vi "VI Konfig LAMBDA.vi"() -> ()   [LabVIEW 2020, in "Lambda_ Komm.lvlib"]
uses:
  Lambda_ Komm.lvlib
  CalGas Aufschaltung/Aufschaltung CalGas_ANZEIGE.ctl
  Visualisierungs Elemente/Auswahlfeld.ctl
  Visualisierungs Elemente/Zahlen-Ausgabefeld.ctl
  CalGas Aufschaltung/FGV CalGas Aktionen.ctl
  FT-IR/FGV FT-IR Gasliste Aktionen.ctl
  FGV Status Lambda Aktionen.ctl
  Messdaten/Aktionen FGV Messdaten.ctl
  FT-IR/FGV FT-IR Parameter.vi
  CalGas Aufschaltung/CalGas Aufschaltung.lvlib
  Grafik/Grafik.lvlib
  FT-IR/FT-IR.lvlib
  Allgemein/allgemeine Sub-VIs.lvlib
  Messdaten/Messdaten.lvlib
panel:
  out "Mwert 3":sgl format="%.1f"
  out "PMwert 3":sgl format="%.1f"
  out "Mwert 2":sgl format="%.3f"
  out "PMwert 2":sgl format="%.3f"
  out "Mwert":sgl format="%.1f"
  out "PMwert":sgl format="%.1f"
  out "A/F Messwertfehler:":bool
  out "O2 Messwertfehler:":bool
  out "Sonden-Innenwiderstand Fehler:":bool
  out "Lambda Messwertfehler:":bool
  out "Kommunikationsfehler:":bool
  out "Sonden-Innenwiderstand:":T1 caption="Ohm" format="%#_5g"
  out "A/F":string
  out "Wert A/F":T1 caption="Konzentration" format="%.1f"
  out "O2":string
  out "Lambda":string
  out "Wert O2":T1 caption="Konzentration" format="%.3f"
  out "Wert Lambda":T1 caption="Konzentration" format="%.1f"
  in  "Aufschaltung CalGas":T2 {"Analysator" items=["FT-IR", "NDIR CO2", "NDIR CO", "PMA", "FID", "CLD"]; "Aufschaltpunkt" items=["über Filterblock", "Analysator direkt", "über Gasteiler", "Gasteiler Eingang"]; "Kalibriergas" items=["Stickstoff", "---", "---", "NOx lo", "NOx hi", "---", "CO2", "CO", "---", "O2", "---", "HC", "---"]}
  out "Graph 3":waveform(dbl)[](graph)
  out "Graph 2":waveform(dbl)[](graph)
  out "Graph1":waveform(dbl)[](graph)
  # "Konfig LAMBDA"
  # "Lambda"
  # "O2"
  # "Luft-Kraftstoff Verhältnis"
  # "Status"
  # "Aufschaltung Kalibriergas"
  # "Kalibriergas"
  # "Aufschaltpunkt"
  # "Analysator"
  # "±"
  # "x"
  # "±"
  # "x"
  # "±"
  # "x"
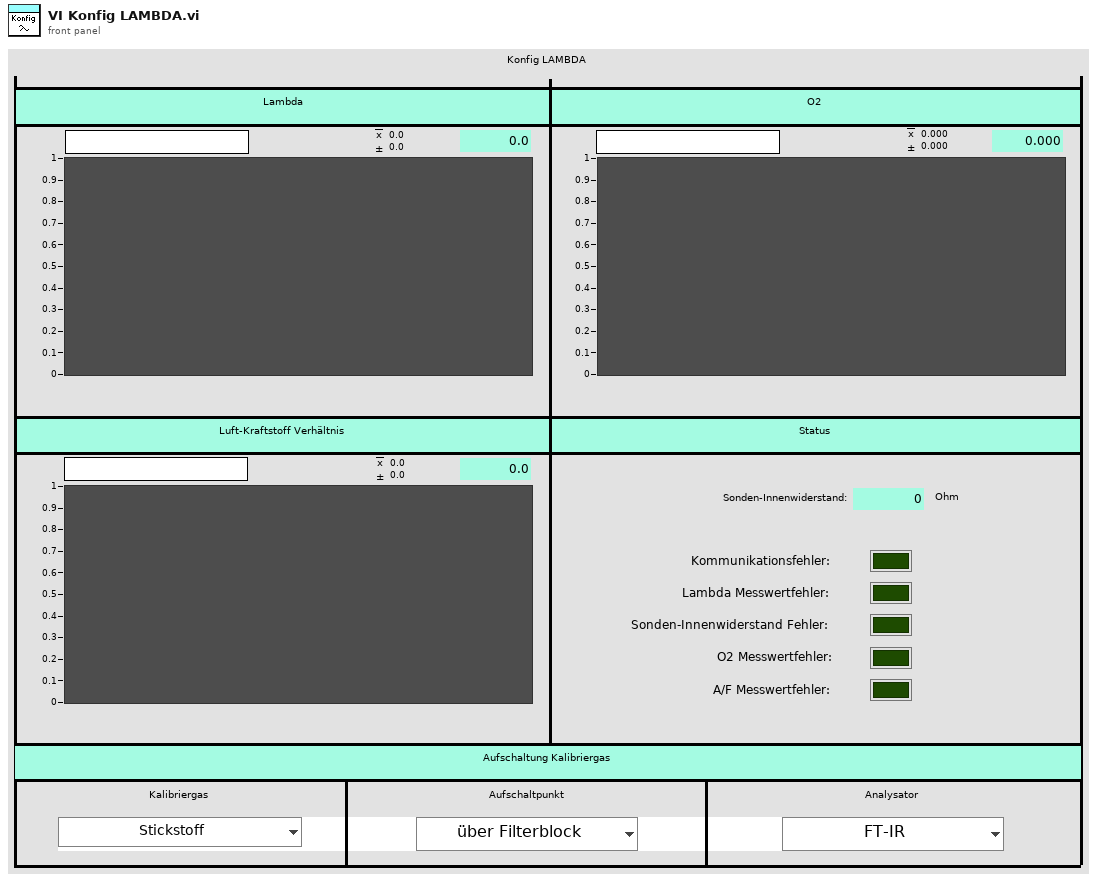
[diagram p1: front panel]
types:
  T1 = typedef "Zahlen-Ausgabefeld.ctl" = sgl
  T2 = typedef "CalGas Aufschaltung.lvlib/Aufschaltung CalGas_ANZEIGE.ctl" = cluster{"Kalibriergas":T3, "Aufschaltpunkt":T3, "Analysator":T3}
  T3 = typedef "Auswahlfeld.ctl" = u16
  T4 = typedef "FT-IR.lvlib/FGV FT-IR Gasliste Aktionen.ctl" = enum16{"lesen", "Gasliste FT-IR", "Gasliste ausgelesen", "laden", "speichern", "löschen"}
  T5 = typedef "CalGas Aufschaltung.lvlib/FGV CalGas Aktionen.ctl" = enum16{"lesen", "Analysator Auswahl", "Def.CalGas", "Aufschaltung CalGas", "laden", "speichern", "KAL extrahieren"}
  T6 = typedef "String - Ausgabefeld.ctl" = string
  T7 = typedef "CalGas Aufschaltung.lvlib/Aufschaltung CalGas.ctl" = cluster{"Kalibriergas":T3, "Aufschaltpunkt":T8, "Analysator":T9}
  T8 = typedef "CalGas Aufschaltung.lvlib/Auswahl Aufschaltpunkt.ctl" = enum16{"über Filterblock", "Analysator direkt", "über PNS", "Entnahme", "Gasdivider"}
  T9 = typedef "CalGas Aufschaltung.lvlib/Auswahl Analysator.ctl" = enum16{"FT-IR", "FID", "PMA", "PMA/FID/FT-IR"}
  T10 = typedef "CalGas Aufschaltung.lvlib/Definition CalGas Anzeige.ctl" = cluster{"Namen":T11, "Werte":T13, "Werte 2":T13, "Einheit":T15, "Messbereiche":T16}
  T11 = typedef "CalGas Aufschaltung.lvlib/CalGas-Namen.ctl" = cluster{"Name":T12, "Name 2":T12, "Name 3":T12, "Name 4":T12, "Name 5":T12, "Name 6":T12, "Name 7":T12, "Name 8":T12, "Name 9":T12, "Name 10":T12, "Name 11":T12, "Name 12":T12}
  T12 = typedef "String - Eingabefeld.ctl" = string
  T13 = typedef "CalGas Aufschaltung.lvlib/CalGas-Werte.ctl" = cluster{"Konzentration 1":T14, "Konzentration 2":T14, "Konzentration 3":T14, "Konzentration 4":T14, "Konzentration 5":T14, "Konzentration 6":T14, "Konzentration 7":T14, "Konzentration 8":T14, "Konzentration 9":T14, "Konzentration 10":T14, "Konzentration 11":T14, "Konzentration 12":T14}
  T14 = typedef "Zahlen-Eingabefeld.ctl" = sgl
  T15 = typedef "CalGas Aufschaltung.lvlib/CalGas-Einheit.ctl" = cluster{"Einheit 1":T3, "Einheit 2":T3, "Einheit 3":T3, "Einheit 4":T3, "Einheit 5":T3, "Einheit 6":T3, "Einheit 7":T3, "Einheit 8":T3, "Einheit 9":T3, "Einheit 10":T3, "Einheit 11":T3, "Einheit 12":T3}
  T16 = typedef "CalGas Aufschaltung.lvlib/CalGas-Messbereiche.ctl" = cluster{"Messbereich 1":T3, "Messbereich 2":T3, "Messbereich 3":T3, "Messbereich 4":T3, "Messbereich 5":T3, "Messbereich 6":T3, "Messbereich 7":T3, "Messbereich 8":T3, "Messbereich 9":T3, "Messbereich 10":T3, "Messbereich 11":T3, "Messbereich 12":T3}
  T17 = typedef "Messdaten.lvlib/Aktionen FGV Messdaten.ctl" = enum16{"lesen", "schreiben", "löschen", "Mittelwerte", "Komponente"}
  T18 = typedef "Lambda_ Komm.lvlib/FGV Status Lambda Aktionen.ctl" = enum16{"lesen", "init", "Istwerte"}
  T19 = typedef "Lambda_ Komm.lvlib/Lambda Fehler.ctl" = cluster{"Komm":bool, "Lambda  Fehler":bool, "Ri Fehler":bool, "O2 Fehler":bool, "A/F Fehler":bool}
  T20 = cluster{"[0]":waveform(dbl), "[1]":waveform(dbl), "[2]":waveform(dbl)}
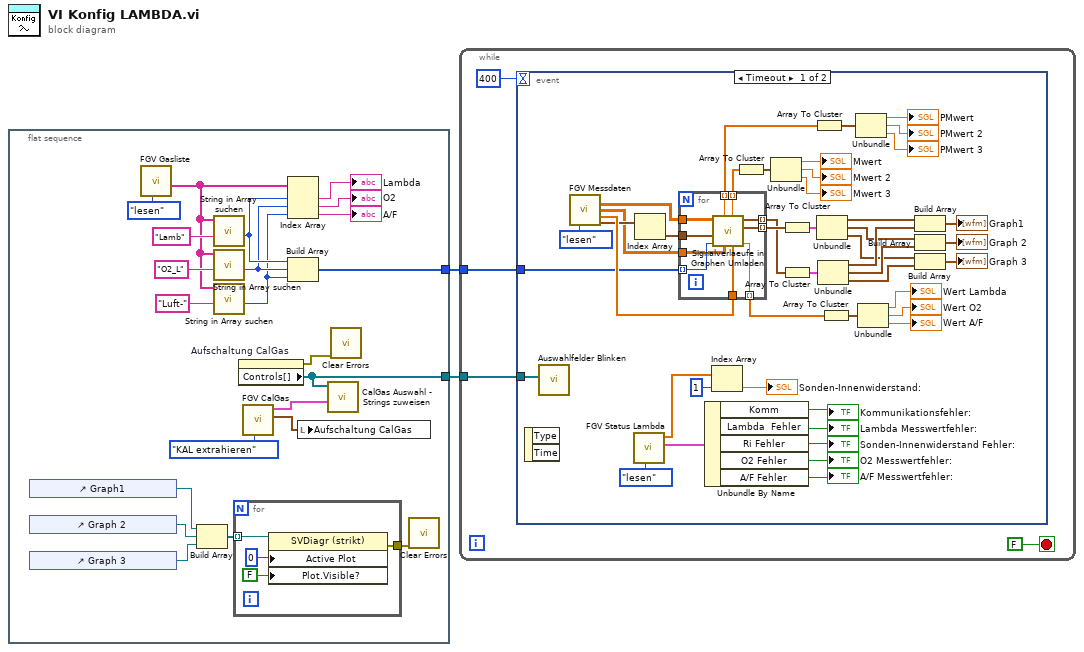
[diagram p0: block diagram]
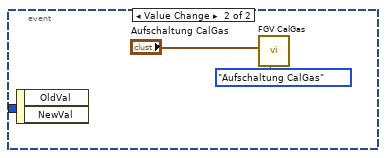
[diagram p2: hidden frame]
diagram:
  n1 = flat-sequence {
    tunnel: [w21] -> w2
    tunnel: [w16] -> w1
    frame #0 {
      n2 = control-ref of="Graph1"() -> (w4:refnum<vi>)
      n3 = control-ref of="Graph 2"() -> (w5:refnum<vi>)
      n4 = control-ref of="Graph 3"() -> (w6:refnum<vi>)
      n5 = call "FGV Gasliste.vi"("Aktionen"=FGV_FT-IR_Gasliste_Aktionen."lesen") -> ("Aktuelle Gasliste gesamt"=w15:T6[])  [unwired: 8 in, 2 out]
      n6 = Build Array(w4, w5, w6) -> (w7:refnum<vi>[])
      n7 = call "String in Array suchen.vi"("Nach String/Zeichen suchen (-)"="Lamb" ("DataSocket:URL"), "String-Array"=w15) -> ("Index"=w14:i32)  [unwired: 7 in, 2 out]
      n8 = call "String in Array suchen.vi"("Nach String/Zeichen suchen (-)"="O2_L" ("DataSocket:URL"), "String-Array"=w15) -> ("Index"=w13:i32)  [unwired: 7 in, 2 out]
      n9 = call "String in Array suchen.vi"("Nach String/Zeichen suchen (-)"="Luft-" ("DataSocket:URL"), "String-Array"=w15) -> ("Index"=w9:i32)  [unwired: 7 in, 2 out]
      n10 = for {
        tunnel: [w26] -> w3
        tunnel: w7 -> [w25] mode=indexing
        n11 = property class="SVDiagr (strikt)"(reference=w25, "Active Plot"=u32 0 ("Aktiver Plot"), "Plot.Visible?"=FALSE ("Plot.Sichtbar")) -> (error out=w26:errorcluster)  [unwired: 1 in, 1 out]
      }
      n12 = property on="Aufschaltung CalGas" class="Cluster (strikt)"() -> (error out=w8:errorcluster, "Controls[]"=w16:refnum<vi>[])  [unwired: 2 in, 1 out]
      n13 = call "FGV CalGas.vi"("Aktionen"=FGV_CalGas_Aktionen."KAL extrahieren") -> ("Aufschaltung CalGas"=w22:T7, "Def.CalGas"=w18:T10)  [unwired: 6 in, 3 out]
      n14 = Index Array(array=w15, index #1=w14, index #2=w13, index #3=w9) -> (element #1=→"Lambda":T6, element #2=→"O2":T6, element #3=→"A/F":T6)
      n15 = Build Array(w14, w13, w9) -> (w21:i32[])
      n16 = local write "Aufschaltung CalGas"(w22) -> ()
      n17 = call "CalGas Auswahl - Strings zuweisen.vi"("Def.CalGas"=w18, "Aufschaltung CalGas"=w16) -> ()  [unwired: 9 in, 1 out]
      n18 = call <vilib>:"Clear Errors.vi"("error in (no error)"=w8) -> ()  [unwired: 5 in, 2 out]
      n19 = call <vilib>:"Clear Errors.vi"("error in (no error)"=w3) -> ()  [unwired: 5 in, 2 out]
    }
  }
  n20 = while {
    tunnel: w2 -> [w30]
    tunnel: w1 -> [w29]
    stop <- FALSE stop-if-true
    n21 = event shown="[0] Timeout" {
      selector: _ -> [_ _]
      dyn-events: _ -> [_ _]
      timeout: 400 -> [_ _]
      tunnel: w30 -> [w37 _]
      tunnel: w29 -> [w78 _]
      event Timeout {
        n22 = event-data() -> ()  [unwired: 1 in, 2 out]
        n23 = call "Auswahlfelder Blinken.vi"("Controls[]"=w78) -> ()  [unwired: 11 in]
        n24 = call "FGV Messdaten.vi"("Aktionen"=Aktionen_FGV_Messdaten."lesen") -> ("Messdaten"=w34:sgl[][], "Mittelwertdaten"=w33:sgl[][], "Deviation"=w41:sgl[], "Zeitstempeln"=w39:timestamp[])  [unwired: 6 in, 5 out]
        n25 = call "FGV Status Lambda.vi"("Aktionen"=FGV_Status_Lambda_Aktionen."lesen") -> ("Lambda Fehler"=w76:T19, "Istwerte"=w74:sgl[])  [unwired: 9 in]
        n26 = Index Array(array=w39) -> (element=w40:timestamp)  [unwired: 1 in]
        n27 = for {
          tunnel: w37 -> [w88] mode=indexing
          tunnel: w34 -> [w87]
          tunnel: w40 -> [w86]
          tunnel: w33 -> [w85]
          tunnel: w41 -> [w84]
          tunnel: [w83] -> w42 mode=indexing
          tunnel: [w82] -> w45 mode=indexing
          tunnel: [w81] -> w44 mode=indexing
          tunnel: [w80] -> w59 mode=indexing
          tunnel: [w79] -> w60 mode=indexing
          n28 = call "Signalverlaeufe in Graphen Umladen.vi"("Deviation"=w84, "Mittelwertdaten"=w85, "Gas-Auswahl"=w88, "t0"=w86, "Werte"=w87) -> ("Konzentration"=w83:sgl, "Mittelwert"=w82:waveform(dbl), "Waveform"=w81:waveform(dbl), "aktuelle Mittelwert"=w80:sgl, "Deviation"=w79:sgl)  [unwired: 2 in]
        }
        n29 = Unbundle By Name(w76) -> ("Komm"=→"Kommunikationsfehler:":bool, "Lambda  Fehler"=→"Lambda Messwertfehler:":bool, "Ri Fehler"=→"Sonden-Innenwiderstand Fehler:":bool, "O2 Fehler"=→"O2 Messwertfehler:":bool, "A/F Fehler"=→"A/F Messwertfehler:":bool)
        n30 = Index Array(array=w74, index=1 ("Index")) -> (element=→"Sonden-Innenwiderstand:":sgl)
        n31 = Array To Cluster(array=w59) -> (cluster=w58:cluster{"[0]":sgl, "[1]":sgl, "[2]":sgl})
        n32 = Unbundle(w58) -> ("[0]"=→"Mwert":sgl, "[1]"=→"Mwert 2":sgl, "[2]"=→"Mwert 3":sgl)
        n33 = Array To Cluster(array=w45) -> (cluster=w47:T20)
        n34 = Array To Cluster(array=w44) -> (cluster=w46:T20)
        n35 = Array To Cluster(array=w60) -> (cluster=w57:cluster{"[0]":sgl, "[1]":sgl, "[2]":sgl})
        n36 = Unbundle(w47) -> ("[0]"=w48:waveform(dbl), "[1]"=w49:waveform(dbl), "[2]"=w50:waveform(dbl))
        n37 = Unbundle(w46) -> ("[0]"=w54:waveform(dbl), "[1]"=w55:waveform(dbl), "[2]"=w56:waveform(dbl))
        n38 = Array To Cluster(array=w42) -> (cluster=w43:cluster{"[0]":sgl, "[1]":sgl, "[2]":sgl})
        n39 = Unbundle(w57) -> ("[0]"=→"PMwert":sgl, "[1]"=→"PMwert 2":sgl, "[2]"=→"PMwert 3":sgl)
        n40 = Unbundle(w43) -> ("[0]"=→"Wert Lambda":sgl, "[1]"=→"Wert O2":sgl, "[2]"=→"Wert A/F":sgl)
        n41 = Build Array(w48, w54) -> (→"Graph1":waveform(dbl)[])
        n42 = Build Array(w49, w55) -> (→"Graph 2":waveform(dbl)[])
        n43 = Build Array(w50, w56) -> (→"Graph 3":waveform(dbl)[])
      }
      event Value Change {
        n44 = event-data() -> ()  [unwired: 1 in, 2 out]
        n45 = call "FGV CalGas.vi"("Aktionen"=FGV_CalGas_Aktionen."Aufschaltung CalGas", "Aufschaltung CalGas"="Aufschaltung CalGas") -> ()  [unwired: 5 in, 5 out]
      }
    }
  }
